vi "FTW-TransferClient-Destroy.vi"(0 "Transfer Client":refnum<class "FTW-TransferClient.lvclass">, 11 "error in":errorcluster) -> (15 "error out":errorcluster)   [LabVIEW 2013, in "FTW-TransferClient.lvclass"]
uses:
  FTW-TransferClient.lvclass
panel:
  # "Inputs"
  # "Outputs"
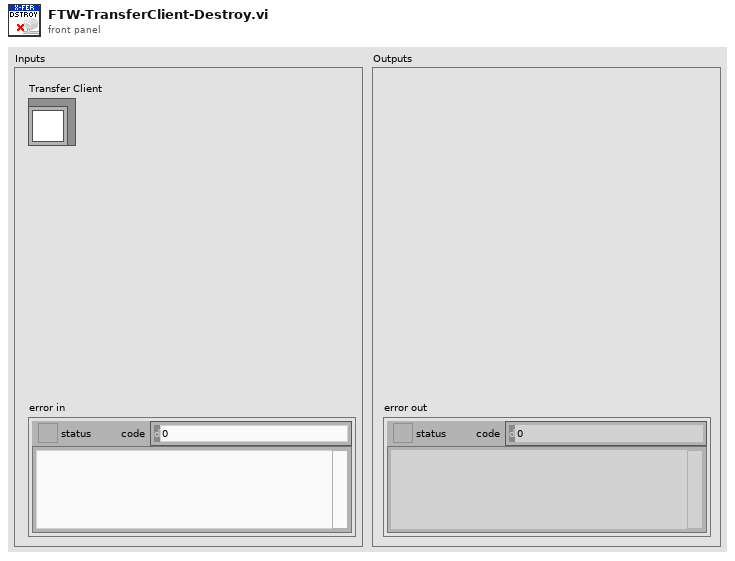
[diagram p1: front panel]
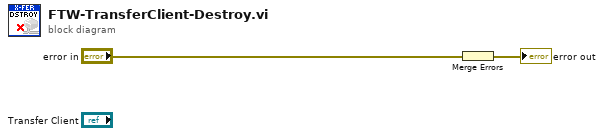
[diagram p0: block diagram]
diagram:
  n1 = Merge Errors("error in") -> (→"error out":errorcluster)
